vi "SendEmailAlert.vi"(6 "UserID,PW":string, 8 "ErrorIn":errorcluster, 9 "Body":string, 10 "Subject":string, 11 "RecipientsIn":string[](array[string])) -> (0 "ErrorOut":errorcluster)   [LabVIEW 2018]
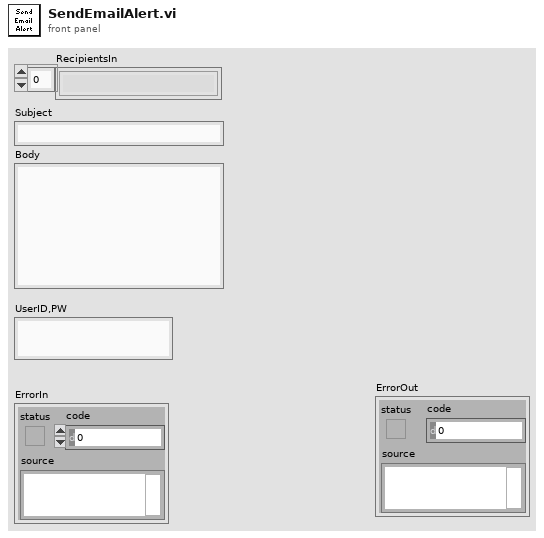
[diagram p1: front panel]
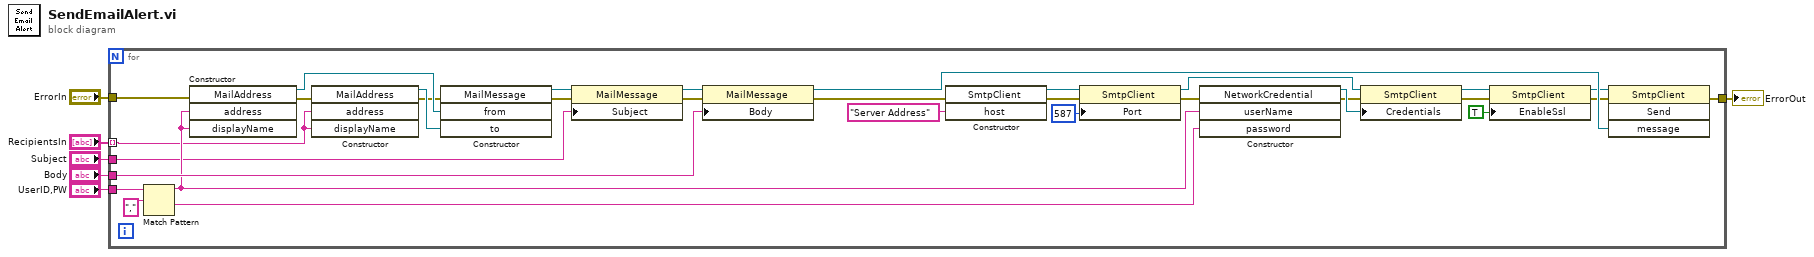
[diagram p0: block diagram]
diagram:
  n1 = for {
    tunnel: "Subject" -> [w7]
    tunnel: "Body" -> [w35]
    tunnel: "ErrorIn" -> [w17]
    tunnel: [w16] -> w3
    tunnel: "UserID,PW" -> [w13]
    tunnel: "RecipientsIn" -> [w9] mode=indexing
    n2 = Match Pattern(string=w13, regular expression=",") -> (before substring=w10:string, after substring=w11:string)  [unwired: 1 in, 2 out]
    n3 = constructor class="MailAddress"(error in=w17, "address"=w10, "displayName"=w10) -> (reference out=w37:refnum<k24>, error out=w20:errorcluster)  [unwired: 2 in, 3 out]
    n4 = constructor class="MailAddress"(error in=w20, "address"=w9, "displayName"=w9) -> (reference out=w38:refnum<k24>, error out=w19:errorcluster)  [unwired: 2 in, 3 out]
    n5 = constructor class="MailMessage"(error in=w19, "from"=w37, "to"=w38) -> (reference out=w25:refnum<k24>, error out=w24:errorcluster)  [unwired: 2 in, 3 out]
    n6 = property class="MailMessage"(reference=w25, error in=w24, "Subject"=w7) -> (reference out=w33:refnum<k24>, error out=w36:errorcluster)
    n7 = property class="MailMessage"(reference=w33, error in=w36, "Body"=w35) -> (reference out=w23:refnum<k24>, error out=w18:errorcluster)
    n8 = constructor class="SmtpClient"(error in=w18, "host"="Server Address" ("Outgoing Mail Server (SMTP)")) -> (reference out=w30:refnum<k24>, error out=w27:errorcluster)  [unwired: 2 in, 2 out]
    n9 = property class="SmtpClient"(reference=w30, error in=w27, "Port"=587) -> (reference out=w29:refnum<k24>, error out=w15:errorcluster)
    n10 = constructor class="NetworkCredential"(error in=w15, "userName"=w10, "password"=w11) -> (reference out=w31:refnum<k24>, error out=w14:errorcluster)  [unwired: 2 in, 3 out]
    n11 = property class="SmtpClient"(reference=w29, error in=w14, "Credentials"=w31) -> (reference out=w28:refnum<k24>, error out=w26:errorcluster)
    n12 = property class="SmtpClient"(reference=w28, error in=w26, "EnableSsl"=TRUE ("Enable SSL")) -> (reference out=w21:refnum<k24>, error out=w22:errorcluster)
    n13 = invoke class="SmtpClient" method="Send"(reference=w21, error in=w22, "message"=w23) -> (error out=w16:errorcluster)  [unwired: 1 in, 3 out]
  }
  "ErrorOut" <- w3
